vi "pythonmaker.vi"(7 "objective":string, 8 "error in":errorcluster, 11 "Table Control":string[][](array[string])) -> (0 "error out":errorcluster)   [LabVIEW 2019]
uses:
  <vilib>/addons/Tools/Unicode/UTF8 Tools.lvlib
panel:
  out "String":string
  out "programme\npython":string
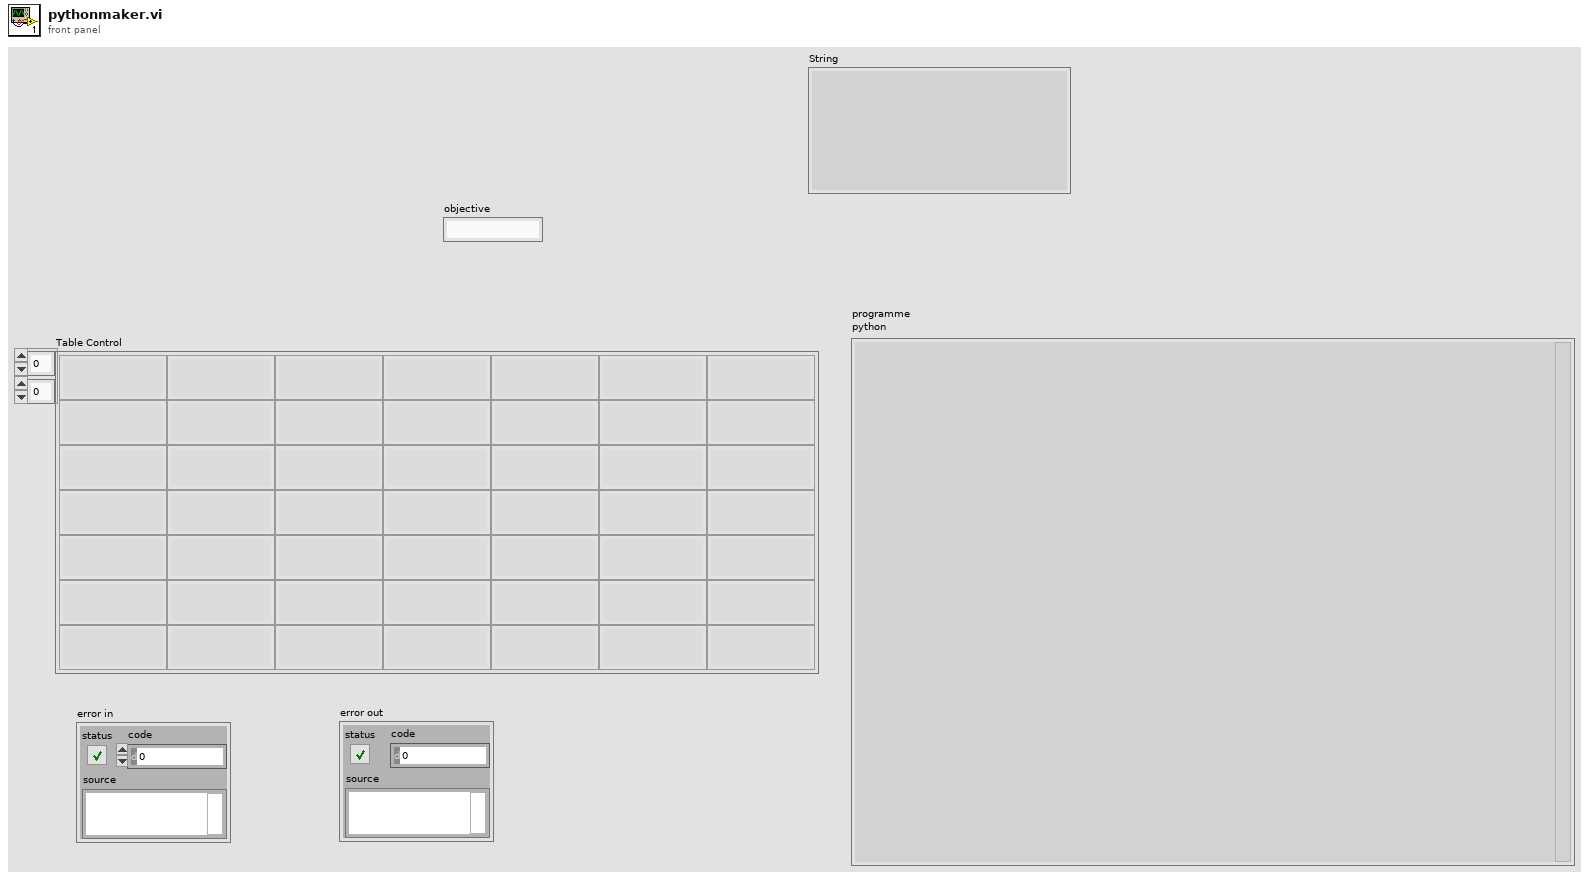
[diagram p1: front panel]
types:
  T1 = enum16{"open", "replace", "create", "open or create", "replace or create", "replace or create with confirmation"}
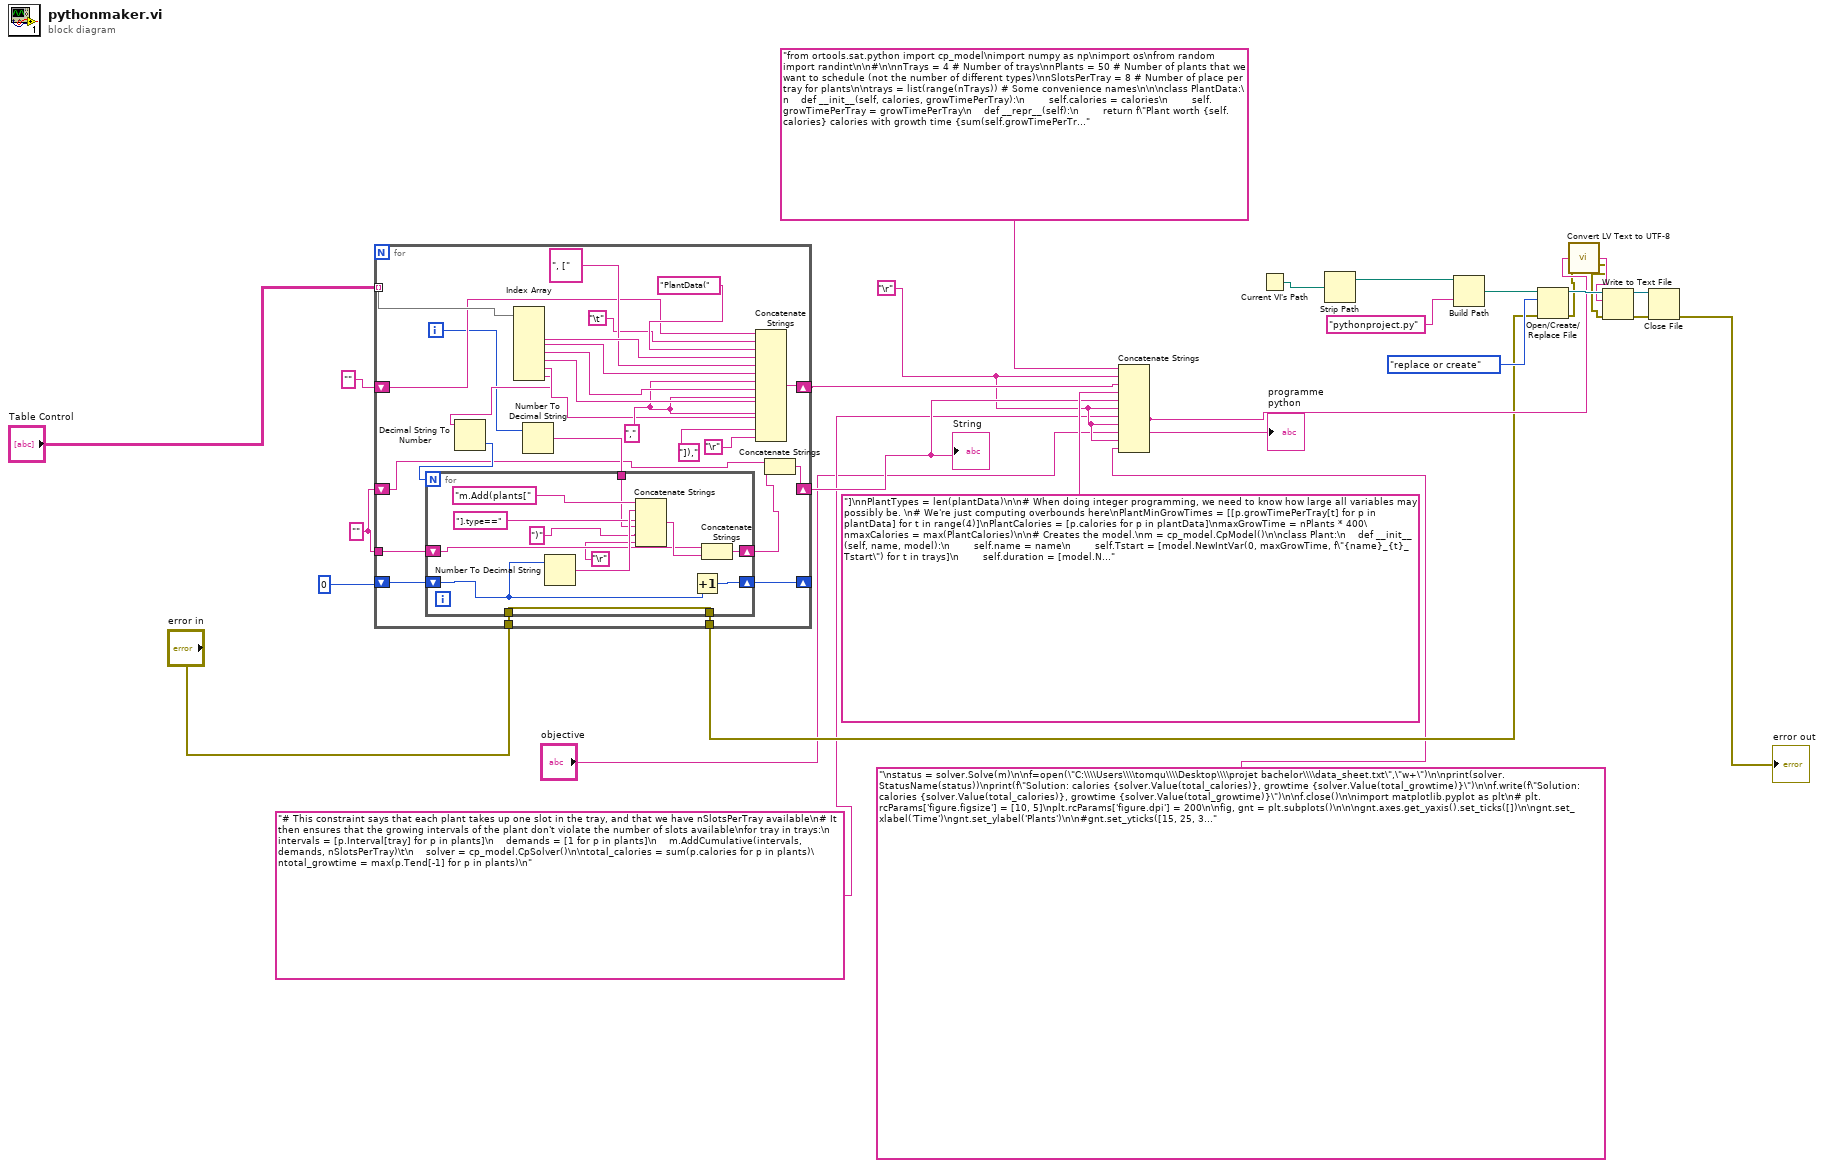
[diagram p0: block diagram]
diagram:
  w7 = ""
  w4 = "\r"
  n1 = for {
    tunnel: "Table Control" -> [w53] mode=indexing
    shift-right: [w33] -> w24
    shift-left: "" -> [w42]
    tunnel: w7 -> [w36]
    tunnel: [w35] -> w9
    tunnel: "error in" -> [w34]
    shift-right: [w30] -> w5
    shift-left: w7 -> [w32]
    shift-right: [w29] -> _
    shift-left: 0 -> [w28]
    i -> [w38]
    w46 = ","
    n2 = Index Array(array=w53) -> (element #2=w51:string, element #3=w49:string, element #4=w48:string, element #5=w47:string, element #6=w45:string, element #7=w40:string)  [unwired: 7 in, 1 out]
    n3 = Decimal String To Number(string=w40) -> (number=w39:i32)  [unwired: 2 in, 1 out]
    n4 = Number To Decimal String(number=w38) -> (decimal integer string=w37:string)  [unwired: 1 in]
    n5 = for {
      N: w39 -> [_]
      shift-right: [w65] -> w29
      shift-left: w28 -> [w62]
      tunnel: w37 -> [w60]
      shift-right: [w58] -> w31
      shift-left: w36 -> [w57]
      tunnel: [w56] -> w35
      tunnel: w34 -> [w56]
      n6 = Number To Decimal String(number=w62) -> (decimal integer string=w64:string)  [unwired: 1 in]
      n7 = Concatenate Strings("m.Add(plants[", w64, "].type==", w60, ")", "\r") -> (w59:string)
      n8 = Increment(x=w62) -> (x+1=w65:i32)
      n9 = Concatenate Strings(w57, w59) -> (w58:string)
    }
    n10 = Concatenate Strings(w42, "\t", "PlantData(", w51, ", [", w49, w46, w48, w46, w47, w46, w45, "]),", "\r") -> (w33:string)
    n11 = Concatenate Strings(w32, w31) -> (w30:string)
  }
  "String" <- w5
  n12 = Concatenate Strings("from ortools.sat.python import cp_model\nimport numpy as np\nimport os\nfrom random import randint\n\n#\n\nnTrays = 4 # Number of trays\nnPlants = 50 # Number of plants that we want to schedule (not the number of different types)\nnSlotsPerTray = 8 # Number of place per tray for plants\n\ntrays = list(range(nTrays)) # Some convenience names\n\n\nclass PlantData:\n    def __init__(self, calories, growTimePerTray):\n        self.calories = calories\n        self.growTimePerTray = growTimePerTray\n    def __repr__(self):\n        return f\"Plant worth {self.calories} calories with growth time {sum(self.growTimePerTray)} (cycle {self.growTimePerTray})\"\n\t\t\n\t\t\n\t\t\n\t\t\n# Specify the data about the types of plants here\n\n# PlantData(calories, [growtime per tray])\nplantData = [", w4, w24, "]\nnPlantTypes = len(plantData)\n\n# When doing integer programming, we need to know how large all variables may possibly be. \n# We're just computing overbounds here\nPlantMinGrowTimes = [[p.growTimePerTray[t] for p in plantData] for t in range(4)]\nPlantCalories = [p.calories for p in plantData]\nmaxGrowTime = nPlants * 400\nmaxCalories = max(PlantCalories)\n\n# Creates the model.\nm = cp_model.CpModel()\n\nclass Plant:\n    def __init__(self, name, model):\n        self.name = name\n        self.Tstart = [model.NewIntVar(0, maxGrowTime, f\"{name}_{t}_Tstart\") for t in trays]\n        self.duration = [model.NewIntVar(0, maxGrowTime, f\"{name}_{t}_duration\") for t in trays]\n        self.Tend = [model.NewIntVar(0, maxGrowTime, f\"{name}_{t}_Tend\") for t in trays]\n        self.Interval = [model.NewIntervalVar(self.Tstart[t], self.duration[t], self.Tend[t], f\"{name}_{t}\") for t in trays]\n        self.minGrowTime = [model.NewIntVar(0, maxGrowTime, f\"{name}_{t}_minGrowTime\") for t in trays]\n        # The type of the plant, from PlantData\n        self.type = model.NewIntVar(0, nPlantTypes, 'type')\n        self.calories = model.NewIntVar(0, maxCalories, f\"{name}_calories\")\n        # Constrain the time in each tray to be long enough\n        for tray, duration in enumerate(self.duration):\n            model.AddElement(self.type, PlantMinGrowTimes[tray], self.minGrowTime[tray])\n            model.Add(self.duration[tray] >= self.minGrowTime[tray])\n        # Go through the trays in order\n        for tray in range(nTrays - 1):\n            model.Add(self.Tstart[tray + 1] == self.Tend[tray])\n        # Calories for this plant\n        model.AddElement(self.type, PlantCalories, self.calories)\n\n# Create the number of requested plant objects\nplants = [Plant(f\"plant_{i}\", m) for i in range(nPlants)]\n", w5, w4, "# This constraint says that each plant takes up one slot in the tray, and that we have nSlotsPerTray available\n# It then ensures that the growing intervals of the plant don't violate the number of slots available\nfor tray in trays:\n    intervals = [p.Interval[tray] for p in plants]\n    demands = [1 for p in plants]\n    m.AddCumulative(intervals, demands, nSlotsPerTray)\t\n    solver = cp_model.CpSolver()\n\ntotal_calories = sum(p.calories for p in plants)\ntotal_growtime = max(p.Tend[-1] for p in plants)\n", w4, "objective", w4, "\nstatus = solver.Solve(m)\n\nf=open(\"C:\\\\Users\\\\tomqu\\\\Desktop\\\\projet bachelor\\\\data_sheet.txt\",\"w+\")\n\nprint(solver.StatusName(status))\nprint(f\"Solution: calories {solver.Value(total_calories)}, growtime {solver.Value(total_growtime)}\")\n\nf.write(f\"Solution: calories {solver.Value(total_calories)}, growtime {solver.Value(total_growtime)}\")\n\nf.close()\n\nimport matplotlib.pyplot as plt\n# plt.rcParams['figure.figsize'] = [10, 5]\nplt.rcParams['figure.dpi'] = 200\n\nfig, gnt = plt.subplots()\n\n\ngnt.axes.get_yaxis().set_ticks([])\n\ngnt.set_xlabel('Time')\ngnt.set_ylabel('Plants')\n\n#gnt.set_yticks([15, 25, 35])\n#gnt.set_yticklabels(['1', '2', '3'])\n\ngnt.grid(True)\n\nheight = 10\ncolors = ('tab:orange', 'tab:blue', 'tab:green', 'tab:red')\nfor p in plants:\n    for t in trays:\n        sched = [(solver.Value(p.Tstart[t]), solver.Value(p.duration[t]))]\n        gnt.broken_barh(sched, (height, 8), facecolors = colors[t])\n    height = height + 10\n\nplt.savefig('C:\\\\Users\\\\tomqu\\\\Desktop\\\\projet bachelor\\\\graphe1.png',format='png')\n\n# Extract the schedule\nschedule = [[[solver.Value(p.Tstart[t]), solver.Value(p.Tend[t])] for t in range(4)] for p in plants]\n\n# Each block is the start and end time for the plant to be in each tray\nemploidutemps=np.array(schedule)\n\n\n\n\ngrowth_time = max(max(max(schedule)))\nnumPlants = np.zeros([growth_time, nTrays])\nfor t in trays:\n    for i in range(growth_time):\n        for p in schedule:\n            if i >= p[t][0] and i < p[t][1]: # The plant is in the tray at this time\n                numPlants[i, t] += 1\n\nfig, gnt = plt.subplots()\n\ngnt.step(range(growth_time), numPlants)\n\ngnt.set_xlabel('Time')\ngnt.set_ylabel('Number of plants in tray')\n\ngnt.grid(True)\n\nplt.savefig('C:\\\\Users\\\\tomqu\\\\Desktop\\\\projet bachelor\\\\graphe2.png',format='png')\n\n# The plant type that each plant chose\nplantTypes = np.array([solver.Value(p.type) for p in plants])\nnumPerType = [sum(plantTypes == i) for i in range(nPlantTypes)]\n\nfig, gnt = plt.subplots()\n\ngnt.bar(range(nPlantTypes), numPerType, 0.35)\ngnt.set_xlabel('Plant Types')\n\nplt.savefig('C:\\\\Users\\\\tomqu\\\\Desktop\\\\projet bachelor\\\\graphe3.png',format='png')\n\nf=open(\"C:\\\\Users\\\\tomqu\\\\Desktop\\\\projet bachelor\\\\données.txt\",\"w+\")\n\nf.write(\"Plantschange=[\")\n\nfor p in plants :\n    f.write(f\"{[solver.Value(p.Tstart[0]), solver.Value(p.Tend[0]), solver.Value(p.Tend[1]), solver.Value(p.Tend[2]), solver.Value(p.Tend[3])]}; \")\n\nf.write(\"]; \\n \")\n\nf.write(f\"Plantsnames={[solver.Value(p.type) for p in plants]}\")\n\nf.write(\";\")\n\nf.close()") -> (w13:string)
  "programme\npython" <- w13
  n13 = Current VI's Path() -> (path=w22:path)
  n14 = Strip Path(path=w22) -> (stripped path=w21:path)  [unwired: 1 out]
  n15 = Build Path(base path=w21, name or relative path="pythonproject.py") -> (appended path=w19:path)
  n16 = Open/Create/Replace File(file path (use dialog)=w19, error in=w9, operation (0:open)=T1."replace or create") -> (refnum out=w17:refnum<file>, error out=w11:errorcluster)  [unwired: 3 in, 1 out]
  n17 = call <vilib>:"Convert LV Text to UTF-8.vi"("LV Text"=w13, "error in"=w11) -> ("UTF-8 Text"=w12:string, "error out"=w10:errorcluster)  [unwired: 12 in]
  n18 = Write to Text File(file (use dialog)=w17, text=w12, error in=w10) -> (refnum out=w15:refnum<file>, error out=w16:errorcluster)  [unwired: 1 in, 1 out]
  n19 = Close File(refnum=w15, error in=w16) -> (error out=→"error out":errorcluster)  [unwired: 1 out]
